vi "Hough Circles.vi"(4 "Hough Circle Parameters (Default: OpenCV Defaults)":T4={"Param1"=100.0, "Param2"=100.0, "Minimum Radius"=0, "Maximum Radius"=0}, 5 "Minimum Distance":dbl=10.0, 6 "Hough Circle Modes (Default: GRADIENT)":T3, 7 "DP":dbl=1.0, 8 "error in (no error)":errorcluster, 11 "Greyscale Image in":T5) -> (0 "error out":errorcluster, 2 "Results":T1[](array[typedef]), 3 "Greyscale Image":T5)   [LabVIEW 2020, in "feature_detection.lvlib"]
doc: "Finds circles in a Greyscale Image using the Hough Transform."
uses:
  feature_detection.lvlib
  image/Greyscale Image.ctl
  Hough Circle Parameters.ctl
  Hough Circle Modes.ctl
  Hough Circle Result.ctl
  common/Image Point (Float).ctl
  Hough Modes.ctl
  common/common.lvlib
  common/bin/gartoolkit_fd_32-1.dll
  image/image.lvlib
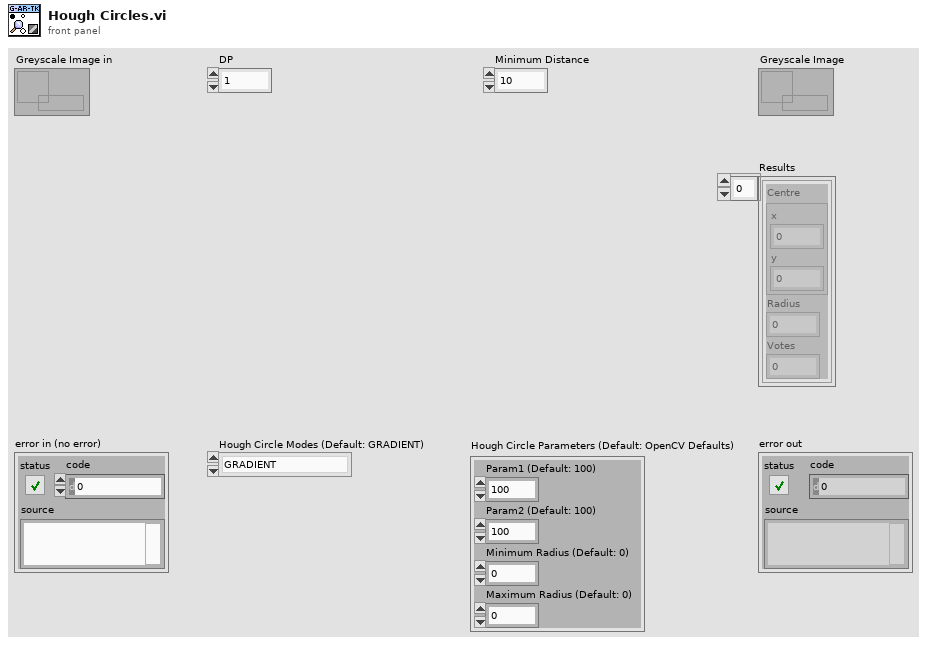
[diagram p1: front panel]
types:
  T1 = typedef "feature_detection.lvlib/Hough Circle Result.ctl" = cluster{"Centre":T2, "Radius":dbl, "Votes":dbl}
  T2 = typedef "common.lvlib/Image Point (Float).ctl" = cluster{"x":dbl, "y":dbl}
  T3 = typedef "feature_detection.lvlib/Hough Circle Modes.ctl" = enum16{"GRADIENT", "GRADIENT_ALT"}
  T4 = typedef "feature_detection.lvlib/Hough Circle Parameters.ctl" = cluster{"Param1":dbl, "Param2":dbl, "Minimum Radius":i32, "Maximum Radius":i32}
  T5 = typedef "image.lvlib/Greyscale Image.ctl" = refnum<data-value>
  T6 = typedef "feature_detection.lvlib/Hough Modes.ctl" = enum16{"STANDARD", "PROBABILISTIC", "MULTI_SCALE", "GRADIENT", "GRADIENT_ALT"}
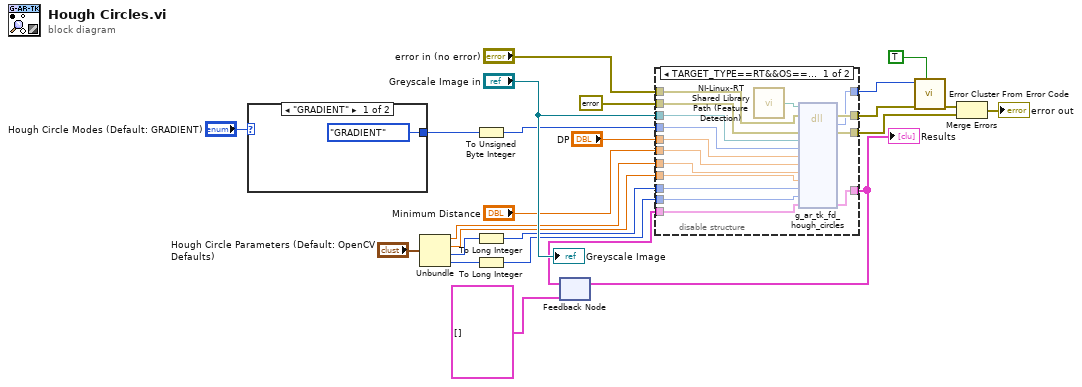
[diagram p0: block diagram]
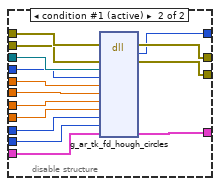
[diagram p2: hidden frame]
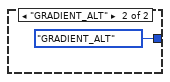
[diagram p3: hidden frame]
diagram:
  n1 = case shown="\"GRADIENT\"" "Hough Circle Modes (Default: GRADIENT)" {
    tunnel: [Hough_Modes."GRADIENT" ("Hough Modes") Hough_Modes."GRADIENT_ALT" ("Hough Modes")] -> w18
    frame "GRADIENT" {
    }
    frame "GRADIENT_ALT" {
    }
  }
  n2 = Unbundle("Hough Circle Parameters (Default: OpenCV Defaults)") -> ("Param1"=w11:dbl, "Param2"=w10:dbl, "Minimum Radius"=w21:i32, "Maximum Radius"=w20:i32)
  n3 = To Unsigned Byte Integer(number=w18) -> (unsigned 8bit integer=w14:u8)
  n4 = To Long Integer(number=w21) -> (32bit integer=w9:i32)
  n5 = To Long Integer(number=w20) -> (32bit integer=w8:i32)
  n6 = feedback #1(T1[] [] ("Array")) -> (w3:T1[])
  n7 = disable-structure shown="TARGET_TYPE==RT&&OS==Linux" {
    disable-tunnel: "error in (no error)" -> [w42 w57]
    disable-tunnel: errorcluster {"status"=FALSE, "code"=0, "source"=""} ("error constant") -> [w41 w56]
    disable-tunnel: "Greyscale Image in" -> [w40 w55]
    disable-tunnel: w14 -> [w39 w54]
    disable-tunnel: "DP" -> [w38 w53]
    disable-tunnel: "Minimum Distance" -> [w37 w52]
    disable-tunnel: w11 -> [w36 w51]
    disable-tunnel: w10 -> [w35 w50]
    disable-tunnel: w9 -> [w34 w49]
    disable-tunnel: w8 -> [w33 w48]
    disable-tunnel: w3 -> [w32 w47]
    disable-tunnel: [w31 w46] -> w7
    disable-tunnel: [w30 w45] -> w6
    disable-tunnel: [w29 w44] -> w5
    disable-tunnel: [w28 w43] -> w4
    frame condition #0 {
      n8 = call "NI-Linux-RT Shared Library Path (Feature Detection).vi"() -> ("Path"=w27:path)
      n9 = dll-call lib="?" fn="g_ar_tk_fd_hough_circles" ("g_ar_toolkit.*.*:g_ar_tk_image_draw_line")(path in=w27, error in=w42, "error_cluster"=w41, "EDVR src"=w40, "hough_mode"=w39, "dp"=w38, "min_distance"=w37, "param1"=w36, "param2"=w35, "min_radius"=w34, "max_radius"=w33, "circles"=w32) -> (error out=w31:errorcluster, w30:i32, "error_cluster"=w29:errorcluster, "circles"=w28:T1[])  [unwired: 9 in, 1 out]
    }
    frame condition #1 (active) {
      n10 = dll-call lib="C:/serenial/lib/g-augmented-reality-toolkit/LabVIEW/common/bin/gartoolkit_fd_*-1.*" fn="g_ar_tk_fd_hough_circles" ("g_ar_toolkit.*.*:g_ar_tk_image_draw_line")(error in=w57, "error_cluster"=w56, "EDVR src"=w55, "hough_mode"=w54, "dp"=w53, "min_distance"=w52, "param1"=w51, "param2"=w50, "min_radius"=w49, "max_radius"=w48, "circles"=w47) -> (error out=w46:errorcluster, w45:i32, "error_cluster"=w44:errorcluster, "circles"=w43:T1[])  [unwired: 10 in, 1 out]
    }
  }
  "Results" <- w4
  n11 = feedback-in #1(w4) -> ()
  n12 = call <vilib>:"Error Cluster From Error Code.vi"("show call chain? (False)"=TRUE, "error in (no error)"=w7, "error code (0)"=w6) -> ("error out"=w23:errorcluster)  [unwired: 6 in]
  n13 = Merge Errors(w23, w5) -> (→"error out":errorcluster)
  "Greyscale Image" <- "Greyscale Image in"
